vi "Iterate.vi"(8 "error in (no error)":errorcluster, 10 "Iterator Settings":T1={"Prepare timeout (ms)"=200, "Iterate timeout (ms)"=50, "Conclude timeout (ms)"=200, "Iterate period (ms)"=200, "Number of iterations"=5, "Time before stop (ms)"=5, "Active Stop Conditions"={"Number of Iterations"=FALSE, "Time Elapsed"=FALSE, "Iteration Result"=FALSE}, "Prepare Msg"=refnum, "Iterate Msg"=refnum, "Conclude Msg"=refnum, "Iterations End Report"=refnum}, 11 "Abstract Iterator Actor in":refnum<class "Abstract Iterator Actor.lvclass">) -> (0 "error out":errorcluster, 3 "Abstract Iterator Actor out":refnum<class "Abstract Iterator Actor.lvclass">)   [LabVIEW 2021, in "Iterator Actor.lvlib" / "Abstract Iterator Actor.lvclass"]
doc: "Iteratively calls the Iterate method of the Client. \nStops the iterations either by receiving the Stop signal, or by any of predefined Stop conditions."
uses:
  Abstract Iterator Actor.lvclass
  Iterator Settings.ctl
  Iterator Actor/Iterator Actor Abstract Messages/Iterator Report Iterations End Msg/Iterator Report Iterations End Msg.lvclass
  <vilib>/ActorFramework/Message/Message.lvclass
  Active Stop Conditions.ctl
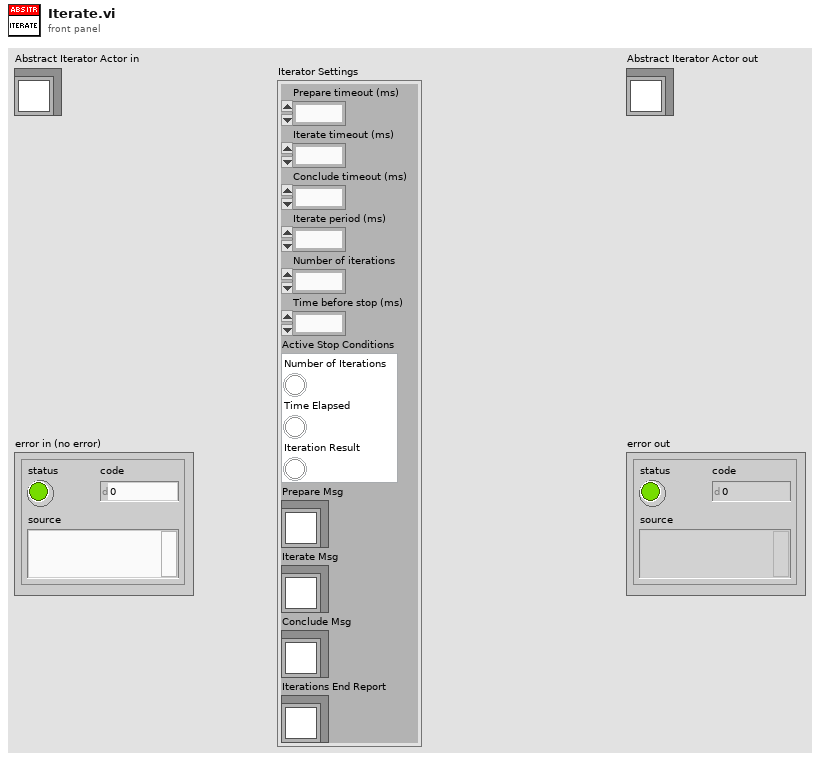
[diagram p1: front panel]
types:
  T1 = typedef "Iterator Actor.lvlib/Abstract Iterator Actor.lvclass/Iterator Settings.ctl" = cluster{"Prepare timeout (ms)":i32, "Iterate timeout (ms)":i32, "Conclude timeout (ms)":i32, "Iterate period (ms)":i32, "Number of iterations":i32, "Time before stop (ms)":i32, "Active Stop Conditions":T2, "Prepare Msg":refnum<class "Message.lvclass">, "Iterate Msg":refnum<class "Message.lvclass">, "Conclude Msg":refnum<class "Message.lvclass">, "Iterations End Report":refnum<class "Iterator Report Iterations End Msg.lvclass">}
  T2 = typedef "Iterator Actor.lvlib/Abstract Iterator Actor.lvclass/Active Stop Conditions.ctl" = cluster{"Number of Iterations":bool, "Time Elapsed":bool, "Iteration Result":bool}
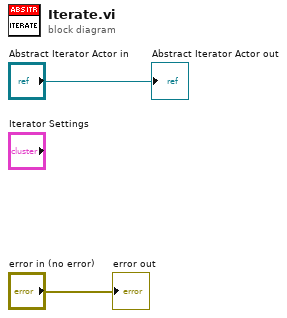
[diagram p0: block diagram]
diagram:
  "error out" <- "error in (no error)"
  "Abstract Iterator Actor out" <- "Abstract Iterator Actor in"
